vi "module-07-exercise-7-2-template.vi"() -> ()   [LabVIEW 2019]
uses:
  <vilib>/Rock Robotics/WPI/ThirdParty/JAS_Junk/TrajLib/Trajectory_Library.lvlib
panel:
  in  "Have Disc \nLimit Switch Sensor":bool
  in  "Battery Voltage":dbl=11.0 min=0.0 max=14.0 step=0.1
  in  "Driver Shoot Button":bool
  in  "Driver Cancel Button":bool
  out "Shoot Request":bool
  out "Digital State Chart":cluster{dbl, dbl, dbl, dbl, dbl, dbl}(graph)
  out "Ready to Shoot":bool
  out "Engage Solenoid":bool
  out "Shooting Motor":bool
  out "State":i32
  out "Current Timer Value":dbl format="%20.3f"
  out "Cur Time":dbl format="%20.3f"
  # "Training Exercise 7-2 Template\nDisc Shooter"
  # "F1"
  # "F2"
  # "F3"
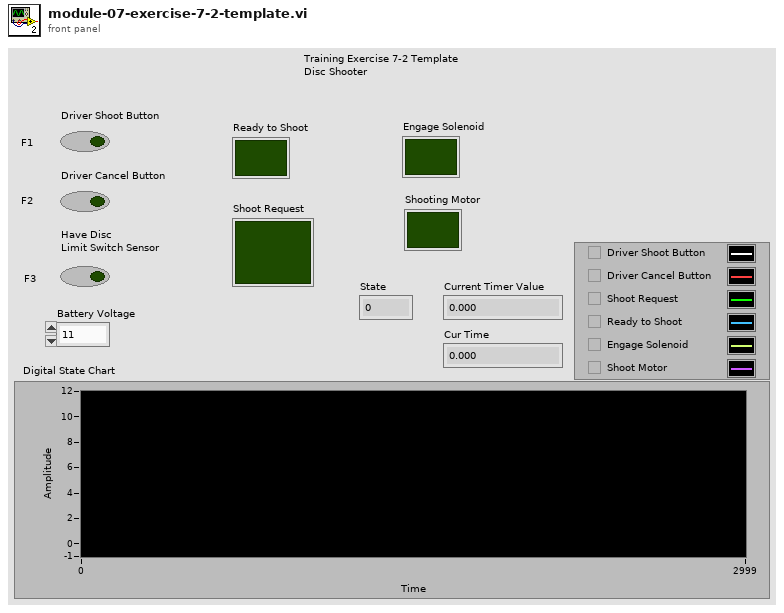
[diagram p1: front panel]
types:
  T1 = typedef "Trajectory_Library.lvlib/TIMER.ctl" = cluster{"StartTime":dbl, "Accumulated TIme":dbl, "Running":bool, "semaphore":T2}
  T2 = typedef "Semaphore RefNum" = refnum<k1>
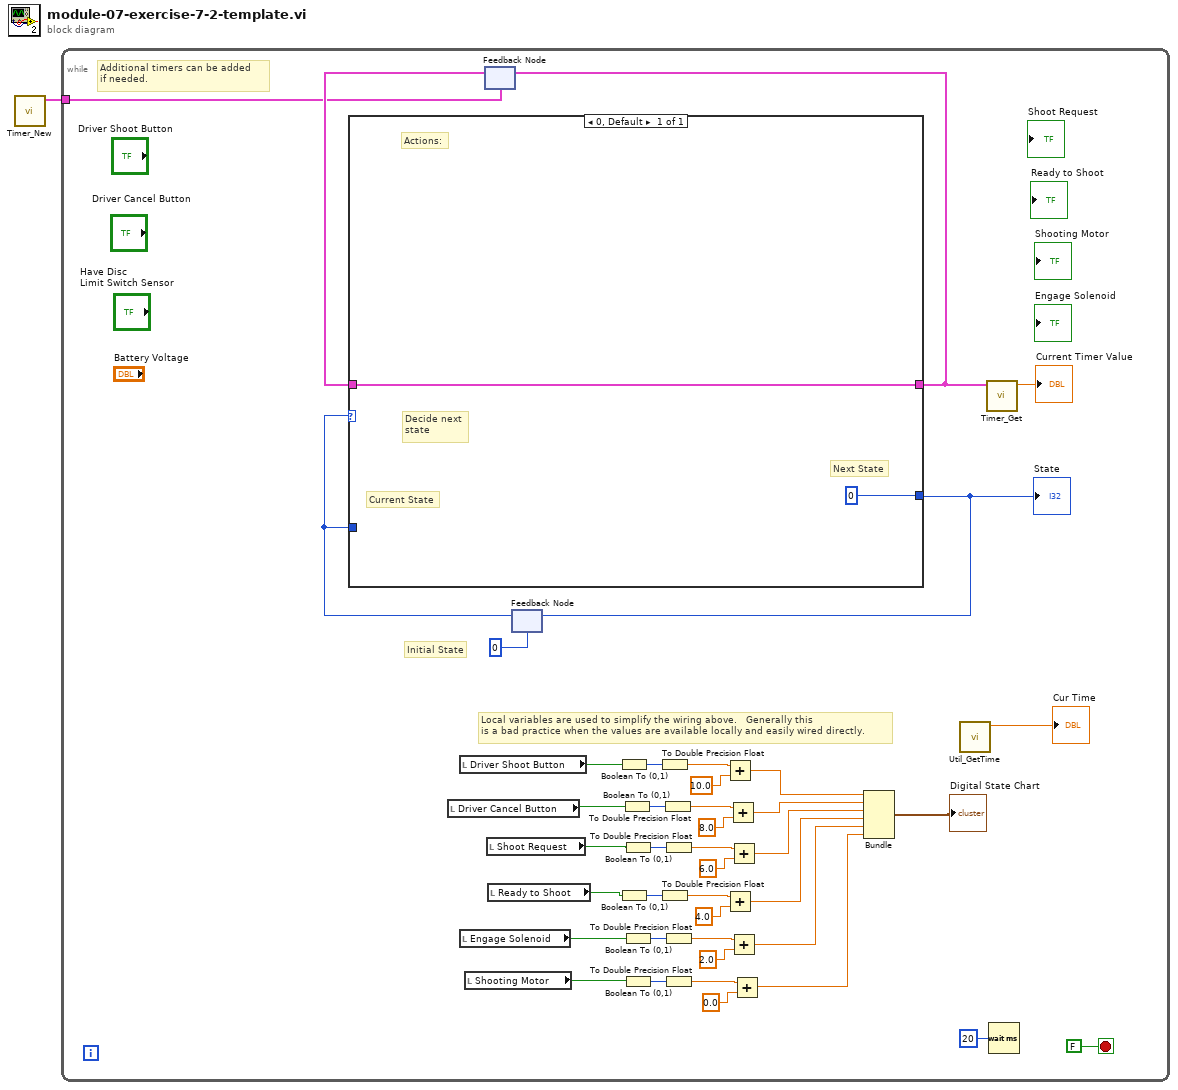
[diagram p0: block diagram]
diagram:
  n1 = call <vilib>:"Timer_New.vi"() -> ("TIMER"=w1:T1)  [unwired: 11 in]
  n2 = while {
    tunnel: w1 -> [w7]
    stop <- FALSE stop-if-true
    # "Additional timers can be added \nif needed."
    # "Initial State"
    # "Local variables are used to simplify the wiring above.   Generally this\nis a bad practice when the values are available locally and easily wired directly."
    n3 = local read "Driver Cancel Button"() -> (w3:bool)
    n4 = local read "Driver Shoot Button"() -> (w2:bool)
    n5 = local read "Engage Solenoid"() -> (w14:bool)
    n6 = local read "Shooting Motor"() -> (w15:bool)
    n7 = feedback #1(w7) -> (w10:T1)
    n8 = local read "Shoot Request"() -> (w13:bool)
    n9 = local read "Ready to Shoot"() -> (w12:bool)
    n10 = feedback #2(u32 0) -> (w9:u32)
    n11 = case shown="0, Default" w9 {
      tunnel: [u32 0] -> w8
      tunnel: [w44] -> w5
      tunnel: w10 -> [w44]
      tunnel: w9 -> [_]
      frame 0, Default {
        # "Decide next\nstate"
        # "Current State"
        # "Next State"
        # "Actions:"
      }
    }
    "State" <- w8
    n12 = feedback-in #1(w5) -> ()
    n13 = feedback-in #2(w8) -> ()
    n14 = Boolean To (0,1)(Boolean=w2) -> (0, 1=w40:i16)
    n15 = Boolean To (0,1)(Boolean=w12) -> (0, 1=w38:i16)
    n16 = Boolean To (0,1)(Boolean=w3) -> (0, 1=w35:i16)
    n17 = Boolean To (0,1)(Boolean=w13) -> (0, 1=w32:i16)
    n18 = Boolean To (0,1)(Boolean=w14) -> (0, 1=w29:i16)
    n19 = Boolean To (0,1)(Boolean=w15) -> (0, 1=w26:i16)
    n20 = To Double Precision Float(number=w40) -> (double precision float=w17:dbl)
    n21 = To Double Precision Float(number=w38) -> (double precision float=w37:dbl)
    n22 = To Double Precision Float(number=w35) -> (double precision float=w34:dbl)
    n23 = To Double Precision Float(number=w32) -> (double precision float=w31:dbl)
    n24 = To Double Precision Float(number=w29) -> (double precision float=w28:dbl)
    n25 = To Double Precision Float(number=w26) -> (double precision float=w25:dbl)
    n26 = Add(x=w17, y=10.0) -> (x+y=w16:dbl)
    n27 = Add(x=w37, y=4.0) -> (x+y=w20:dbl)
    n28 = Add(x=w34, y=8.0) -> (x+y=w22:dbl)
    n29 = Add(x=w31, y=6.0) -> (x+y=w21:dbl)
    n30 = Add(x=w28, y=2.0) -> (x+y=w24:dbl)
    n31 = Add(x=w25, y=0.0) -> (x+y=w23:dbl)
    n32 = Bundle(w16, w22, w21, w20, w24, w23) -> (→"Digital State Chart":cluster{dbl, dbl, dbl, dbl, dbl, dbl})  [unwired: 1 in]
    n33 = call <vilib>:"Util_GetTime.vi"() -> ("FPGA_Time_Seconds"=→"Cur Time":dbl)  [unwired: 10 in, 1 out]
    n34 = call <vilib>:"Timer_Get.vi"("TIMER"=w5) -> ("CurrentTImer"=→"Current Timer Value":dbl)  [unwired: 10 in]
    n35 = Wait (ms)(milliseconds to wait=u32 20) -> ()  [unwired: 1 out]
  }
